vi "MyDerivativePoly.vi"(2 "n-diff":i32 caption="number of points\nto differentiate over", 3 "data Array":dbl[](array[numeric]), 4 "time Array":dbl[](array[numeric]), 5 "Interpolation Order":dbl=nan) -> (0 "2nd Derivative":dbl, 1 "1st Derivative":dbl)   [LabVIEW 2025]
uses:
  <vilib>/Analysis/polynomials.llb/Scalar Polynomial Evaluation (DBL).vi
  <vilib>/Analysis/NI_AALPro.lvlib
panel:
  out "Offset":i32
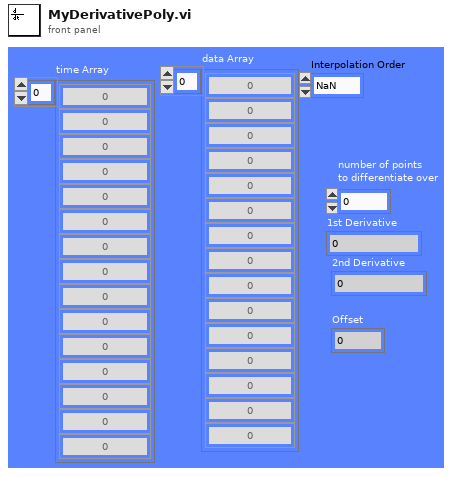
[diagram p1: front panel]
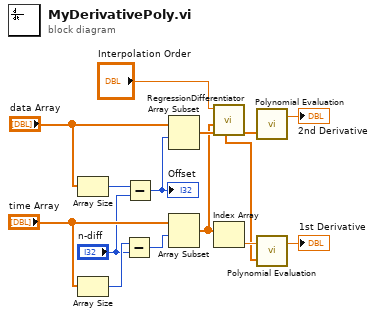
[diagram p0: block diagram]
diagram:
  n1 = Array Size(array="data Array") -> (size(s)=w12:i32)
  n2 = Array Size(array="time Array") -> (size(s)=w13:i32)
  n3 = Subtract(x=w13, y="n-diff") -> (x-y=w10:i32)
  n4 = Subtract(x=w12, y="n-diff") -> (x-y=w9:i32)
  "Offset" <- w9
  n5 = Array Subset(array="data Array", index=w9) -> (w8:dbl[])  [unwired: 1 in]
  n6 = Array Subset(array="time Array", index=w10) -> (w7:dbl[])  [unwired: 1 in]
  n7 = call "RegressionDifferentiator.vi"("y"=w8, "x"=w7, "Interpolation Order"="Interpolation Order") -> ("P''(x)"=w2:dbl[], "P'(x)"=w3:dbl[])  [unwired: 3 in, 4 out]
  n8 = Index Array(array=w7) -> (element=w6:dbl)  [unwired: 1 in]
  n9 = call-poly <vilib>:"Polynomial Evaluation.vi"("P(x)"=w2) -> ("P(a)"=→"2nd Derivative":dbl)  [unwired: 1 in, 1 out]
  n10 = call-poly <vilib>:"Polynomial Evaluation.vi"("P(x)"=w3, "a"=w6) -> ("P(a)"=→"1st Derivative":dbl)  [unwired: 1 out]
